vi "_FPGA_StepwiseScan_StepController.vi"(8 "FirstConj":bool, 9 "Init":bool, 10 "Conj_strobe_in":bool, 11 "StepwiseScan.#ConjForAStep":u8) -> (0 "Start?_strobe":bool, 2 "ToNextStep":bool)   [LabVIEW 2018]
uses:
  <instrlib>/_niInstr/Basic Elements/v1/FPGA/niInstr Basic Elements v1 FPGA.lvlib
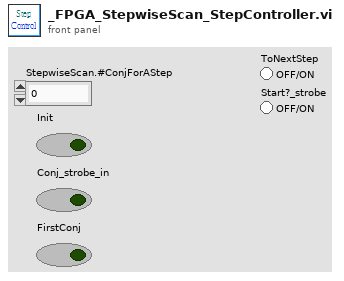
[diagram p1: front panel]
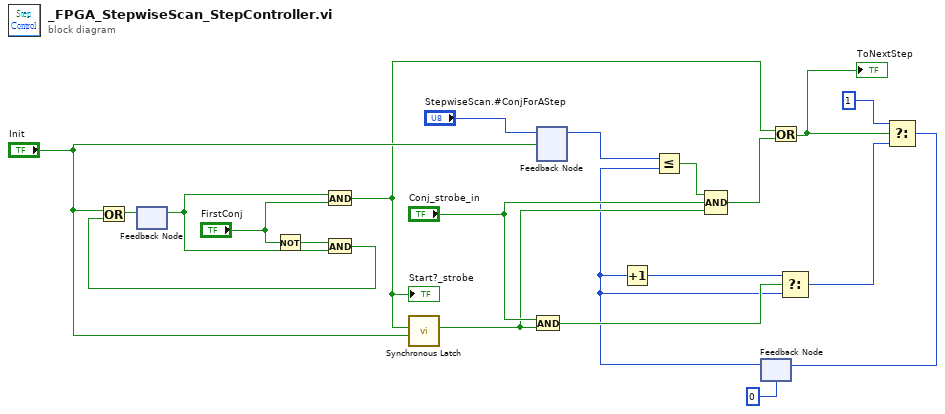
[diagram p0: block diagram]
diagram:
  n1 = feedback #1() -> (w14:bool)  [unwired: 1 in]
  n2 = Not(x="FirstConj") -> (.not. x?=w16:bool)
  n3 = And(x=w14, y="FirstConj") -> (x .and. y?=w4:bool)
  "Start?_strobe" <- w4
  n4 = And(x=w16, y=w14) -> (x .and. y?=w13:bool)
  n5 = Or(x="Init", y=w13) -> (x .or. y?=w15:bool)
  n6 = feedback-in #1(w15) -> ()
  n7 = call <instrlib>:"Synchronous Latch.vi"("clear"="Init", "set"=w4) -> ("out"=w6:bool)  [unwired: 9 in]
  n8 = And(x="Conj_strobe_in", y=w6) -> (x .and. y?=w11:bool)
  n9 = feedback-in #2("StepwiseScan.#ConjForAStep", "Init") -> ()
  n10 = feedback #2() -> (w9:u8)  [unwired: 1 in]
  n11 = feedback #3(u8 0 ("StepwiseScan.#ConjForStep")) -> (w1:u8)
  n12 = Increment(x=w1) -> (x+1=w2:u8)
  n13 = Less Or Equal?(x=w9, y=w1) -> (x <= y?=w10:bool)
  n14 = Compound Arithmetic op=AND(w10, "Conj_strobe_in", w6) -> (w5:bool)
  n15 = Or(x=w4, y=w5) -> (x .or. y?=w3:bool)
  "ToNextStep" <- w3
  n16 = Select(t=w2, s=w11, f=w1) -> (s? t:f=w8:u8)
  n17 = Select(t=u8 1 ("StepwiseScan.#ConjForStep"), s=w3, f=w8) -> (s? t:f=w18:u8)
  n18 = feedback-in #3(w18) -> ()
